vi "get encoder pos.vi"(8 "error in (no error)":errorcluster, 11 "ch":i32) -> (0 "error out":errorcluster, 3 "function return":i32)   [LabVIEW 2014, in "libroboticscape.lvlib"]
doc: "int get_encoder_pos(int ch);"
uses:
  libroboticscape.lvlib
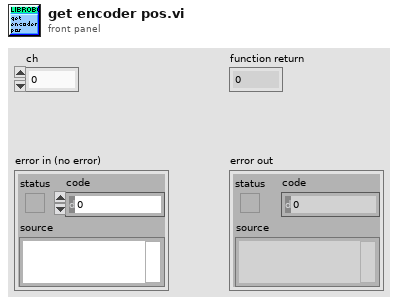
[diagram p1: front panel]
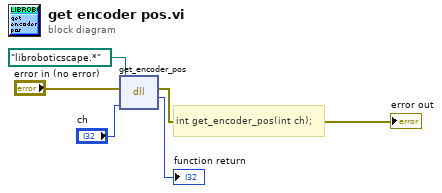
[diagram p0: block diagram]
diagram:
  # "int get_encoder_pos(int ch);"
  n1 = dll-call lib="C:/Users/ktalke/Documents/Jessie Build/Libroboticscape/libroboticscape.so" fn="get_encoder_pos"(path in=path "libroboticscape.*", error in="error in (no error)", "ch"="ch") -> (error out=→"error out":errorcluster, "return type"=→"function return":i32)  [unwired: 2 in, 1 out]
